vi "ShowOperatorPane.vi"(8 "error in (no error)":errorcluster, 10 "Visible":bool, 11 "GUI_Handler_Main in":refnum<class "GUI_Handler_Main.lvclass">) -> (0 "error out":errorcluster, 3 "GUI_Handler_Main out":refnum<class "GUI_Handler_Main.lvclass">)   [LabVIEW 2017, in "GUI_Handler_Main.lvclass"]
uses:
  GUI_Handler_Main.lvclass
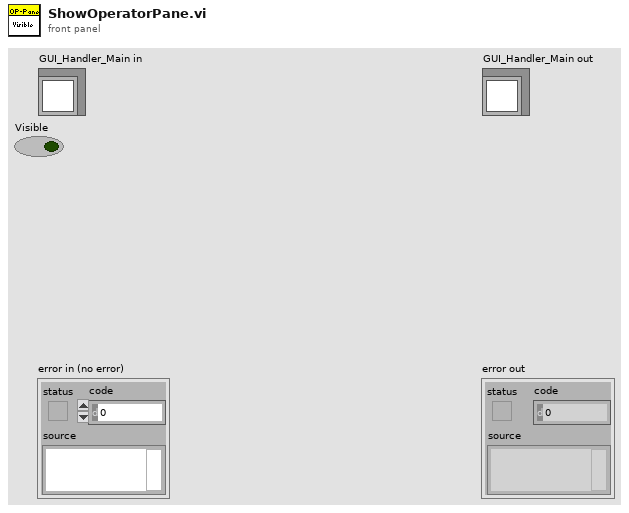
[diagram p1: front panel]
types:
  T1 = cluster{"Start Alt":refnum<vi>, "Stop":refnum<vi>, "Operatør beskeder":refnum<vi>}
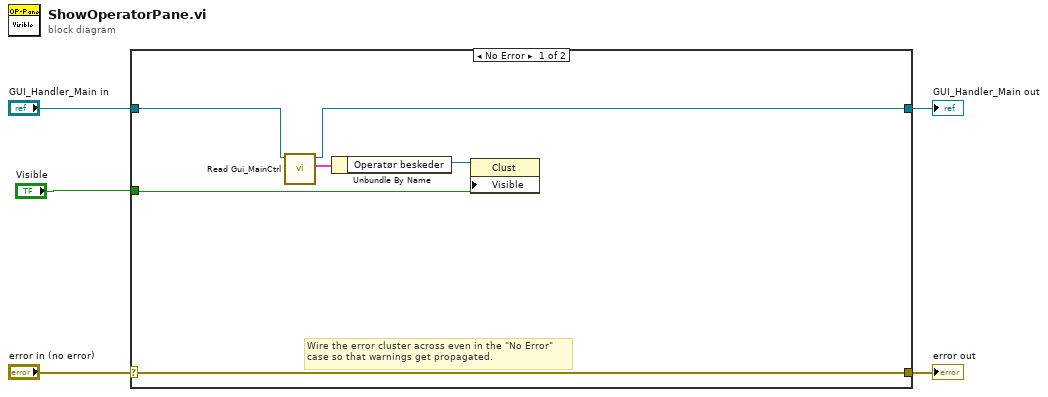
[diagram p0: block diagram]
diagram:
  n1 = case shown="No Error" "error in (no error)" {
    selector: "error in (no error)" -> [w11 w13]
    tunnel: [w11 w13] -> w4
    tunnel: [w9 w12] -> w2
    tunnel: "GUI_Handler_Main in" -> [w10 w12]
    tunnel: "Visible" -> [w6 _]
    frame No Error {
      # "Wire the error cluster across even in the \"No Error\"\ncase so that warnings get propagated."
      n2 = call-dynamic "Read Gui_MainCtrl.vi"("GUI_Handler_Main in"=w10) -> ("Gui_MainCtrl"=w8:T1, "GUI_Handler_Main out"=w9:refnum<class "GUI_Handler_Main.lvclass">)  [unwired: 8 in, 1 out]
      n3 = Unbundle By Name(w8) -> ("Operatør beskeder"=w7:refnum<vi>)
      n4 = property class="Clust"(reference=w7, "Visible"=w6) -> ()  [unwired: 1 in, 2 out]
    }
    frame Error {
    }
  }
  "error out" <- w4
  "GUI_Handler_Main out" <- w2
